vi "save.vi"(8 "error in (no error)":errorcluster, 11 "_data in":refnum<class "_data.lvclass">) -> (0 "error out":errorcluster, 3 "_data out":refnum<class "_data.lvclass">)   [LabVIEW 2019, in "_data.lvlib" / "_data.lvclass"]
uses:
  _data.lvclass
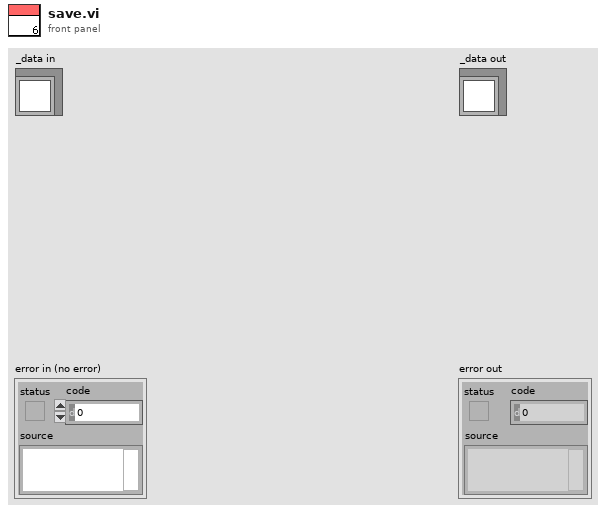
[diagram p1: front panel]
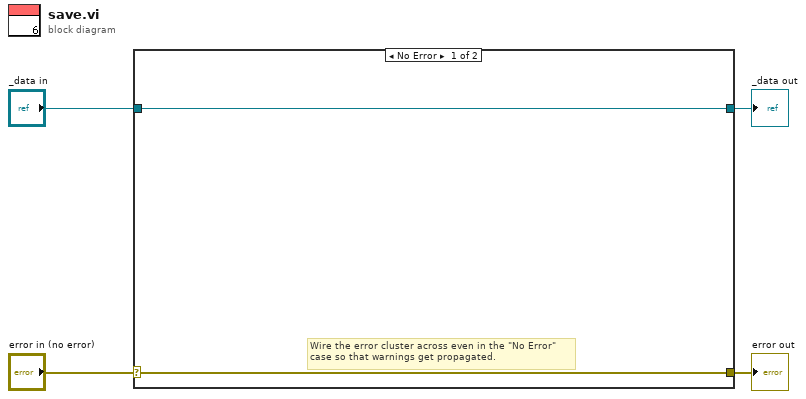
[diagram p0: block diagram]
diagram:
  n1 = case shown="No Error" "error in (no error)" {
    selector: "error in (no error)" -> [w5 w8]
    tunnel: [w5 w8] -> w3
    tunnel: [w6 w7] -> w1
    tunnel: "_data in" -> [w6 w7]
    frame No Error {
      # "Wire the error cluster across even in the \"No Error\"\ncase so that warnings get propagated."
    }
    frame Error {
    }
  }
  "error out" <- w3
  "_data out" <- w1
